vi "getFPGAReference.vi"(11 "FPGATelemetry in":refnum<class "FPGATelemetry.lvclass">) -> (2 "FPGAReference":refnum<k20>, 3 "FPGATelemetry out":refnum<class "FPGATelemetry.lvclass">)   [LabVIEW 2015, in "FPGATelemetry.lvclass"]
uses:
  FPGATelemetry.lvclass
  FPGATelemetry.lvclass/FPGATelemetry.ctl
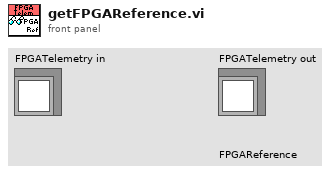
[diagram p1: front panel]
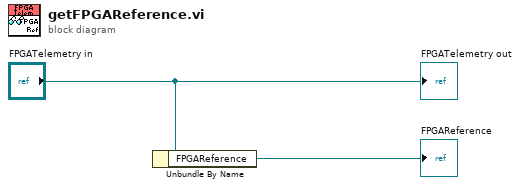
[diagram p0: block diagram]
diagram:
  n1 = Unbundle By Name("FPGATelemetry in") -> ("FPGAReference"=→"FPGAReference":refnum<k20>)
  "FPGATelemetry out" <- "FPGATelemetry in"
